vi "libssh2_sftp_fstat.vi"(8 "error in (no error)":errorcluster, 11 "sftp handle":T2) -> (0 "error out":errorcluster, 2 "attributes out":T1)   [LabVIEW 2013, in "libssh2.lvlib"]
doc: "Get the attributes of a file handle."
uses:
  libssh2.lvlib
  SFTP Handle Refnum.ctl
  libssh2_sftp_attributes.ctl
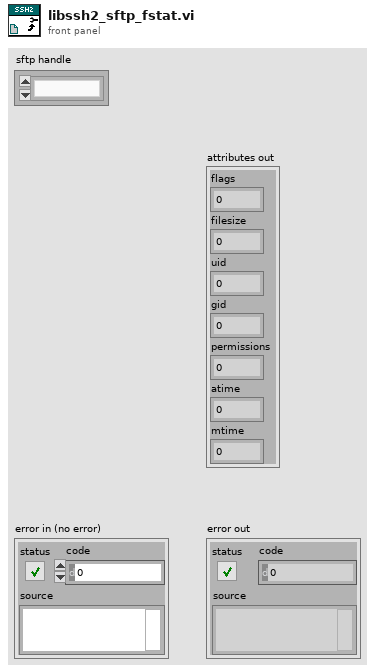
[diagram p1: front panel]
types:
  T1 = typedef "libssh2.lvlib/libssh2_sftp_attributes.ctl" = cluster{"flags":u32, "filesize":u64, "uid":u32, "gid":u32, "permissions":u32, "atime":u32, "mtime":u32}
  T2 = typedef "libssh2.lvlib/SFTP Handle Refnum.ctl" = refnum<k1>
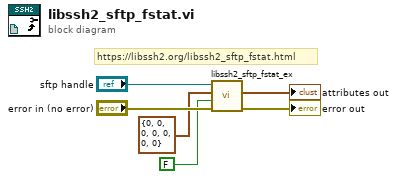
[diagram p0: block diagram]
diagram:
  # "https://libssh2.org/libssh2_sftp_fstat.html"
  n1 = call "libssh2_sftp_fstat_ex.vi"("error in (no error)"="error in (no error)", "set"=FALSE, "attributes in"=T1 {"flags"=0, "filesize"=0, "uid"=0, "gid"=0, "permissions"=0, "atime"=0, "mtime"=0} ("attributes"), "sftp handle"="sftp handle") -> ("error out"=→"error out":errorcluster, "attributes out"=→"attributes out":T1)  [unwired: 6 in]
